vi "2100_Select_Run Script_Reconfigure for Waveform_HSDIO.vi"(7 "max time milliseconds (10 seconds)":i32=10000, 8 "error in (no error)":errorcluster, 9 "Script_Subname":string="Burnin46V", 10 "USID":T1 max=15 format="%.0x", 11 "Semiconductor Module Context":T2) -> (0 "error out":errorcluster)   [LabVIEW 2013]
uses:
  <vilib>/NI_TestStand_SemiconductorModule/NI_TestStand_Semiconductor_Module.lvlibp/PinMap/General/SemiconductorModuleContext.ctl
  Controls/USID.ctl
  <instrlib>/niHSDIO/niHSDIO.llb/niHSDIO_ctl Generation Mode Values (Ring).ctl
  <vilib>/NI_TestStand_SemiconductorModule/NI_TestStand_Semiconductor_Module.lvlibp
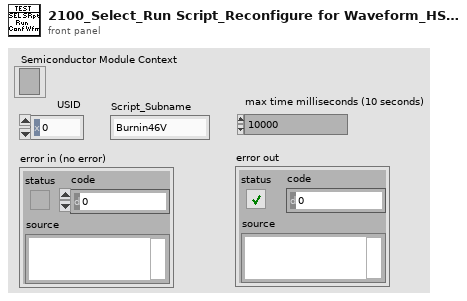
[diagram p1: front panel]
types:
  T1 = typedef "USID.ctl" = u8
  T2 = typedef "NI_TestStand_Semiconductor_Module.lvlibp/SemiconductorModuleContext.ctl" = refnum<k7>
  T3 = typedef "niHSDIO_ctl Generation Mode Values (Ring).ctl" = i32
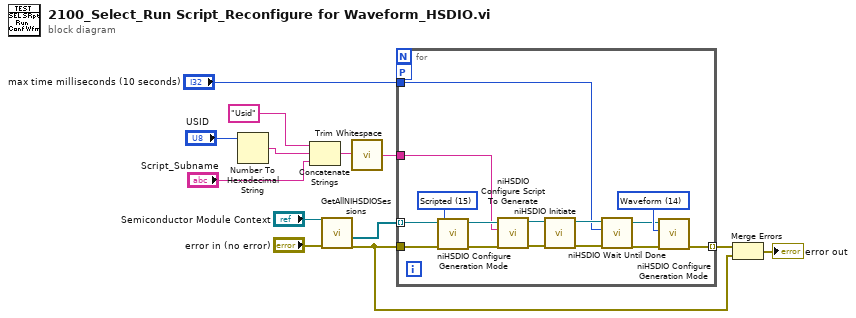
[diagram p0: block diagram]
diagram:
  n1 = Number To Hexadecimal String(2:"USID") -> (0:w3:string)  [unwired: 1 in]
  n2 = Concatenate Strings("Usid" ("string"), w3, "Script_Subname") -> (w2:string)
  n3 = call <vilib>:"GetAllNIHSDIOSessions.vi"("error in (no error)"="error in (no error)", "Semiconductor Module Context"="Semiconductor Module Context") -> ("error out"=w7:errorcluster, "Generation Sessions"=w10:refnum<k15>[])  [unwired: 6 in, 2 out]
  n4 = call <vilib>:"Trim Whitespace.vi"("string"=w2) -> ("trimmed string"=w1:string)  [unwired: 1 in]
  n5 = for {
    tunnel: "max time milliseconds (10 seconds)" -> [w18]
    tunnel: w1 -> [w17]
    tunnel: w7 -> [w16]
    tunnel: w10 -> [w15] mode=indexing
    workers-P: _ -> [_]
    tunnel: [w14] -> w9 mode=indexing
    w27 = T3 14 items=["Waveform"=14, "Scripted"=15] ("generation mode (waveform)")
    w28 = T3 15 items=["Waveform"=14, "Scripted"=15] ("generation mode (waveform)")
    n6 = call <instrlib>:"niHSDIO Configure Generation Mode.vi"("error in (no error)"=w16, "generation mode (waveform)"=w28, "instrument handle"=w15) -> ("error out"=w20:errorcluster, "instrument handle out"=w19:refnum<k15>)  [unwired: 7 in]
    n7 = call <instrlib>:"niHSDIO Configure Script To Generate.vi"("error in (no error)"=w20, "script name"=w17, "instrument handle"=w19) -> ("error out"=w23:errorcluster, "instrument handle out"=w24:refnum<k15>)  [unwired: 7 in]
    n8 = call <instrlib>:"niHSDIO Initiate.vi"("error in (no error)"=w23, "instrument handle"=w24) -> ("error out"=w26:errorcluster, "instrument handle out"=w25:refnum<k15>)  [unwired: 8 in]
    n9 = call <instrlib>:"niHSDIO Wait Until Done.vi"("error in (no error)"=w26, "max time milliseconds (10 seconds)"=w18, "instrument handle"=w25) -> ("error out"=w22:errorcluster, "instrument handle out"=w21:refnum<k15>)  [unwired: 7 in]
    n10 = call <instrlib>:"niHSDIO Configure Generation Mode.vi"("error in (no error)"=w22, "generation mode (waveform)"=w27, "instrument handle"=w21) -> ("error out"=w14:errorcluster)  [unwired: 7 in, 1 out]
  }
  n11 = Merge Errors(w9, w7) -> (→"error out":errorcluster)
